vi "DAC Save Results.vi"(8 "error in":errorcluster, 9 "Log Details?":bool, 10 "tdms file":refnum<k34>, 11 "DAC Traverse in":refnum<class "DAC Traverse.lvclass">) -> (0 "error out":errorcluster)   [LabVIEW 2019, in "DAC.lvlib" / "DAC Traverse.lvclass"]
uses:
  DAC Traverse.lvclass
  DAC.lvclass
  C:/Users/krio/Documents/LV_Projects/test-stand/App/DAC/DAC.lvclass
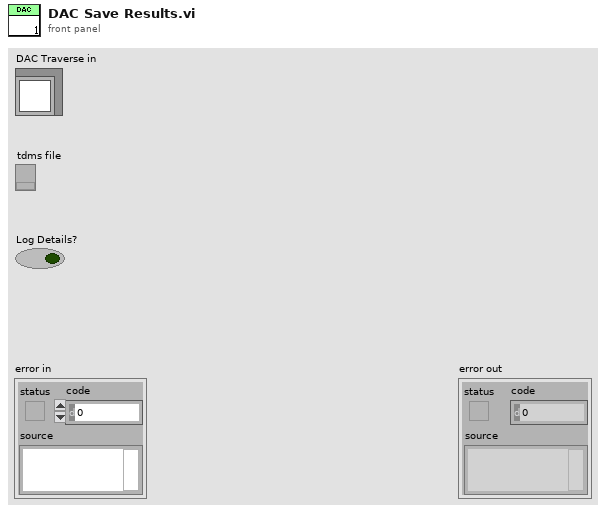
[diagram p1: front panel]
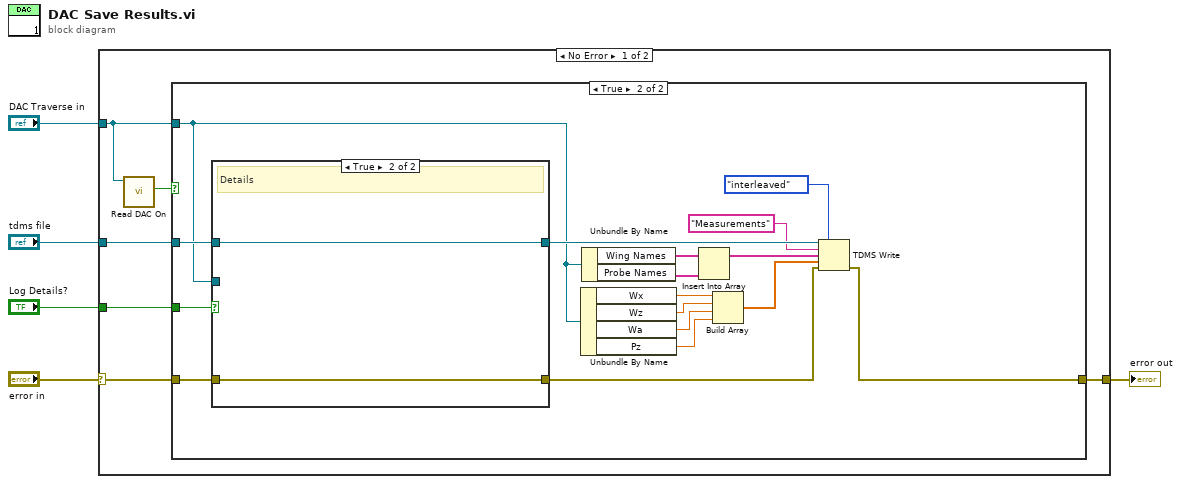
[diagram p0: block diagram]
diagram:
  n1 = case shown="No Error" "error in" {
    selector: "error in" -> [w6 w34]
    tunnel: "DAC Traverse in" -> [w11 _]
    tunnel: "tdms file" -> [w9 _]
    tunnel: [w8 w34] -> w2
    tunnel: "Log Details?" -> [w7 _]
    frame No Error {
      n2 = call "Read DAC On.vi"("DAC in"=w11) -> ("DAC On"=w10:bool)  [unwired: 8 in, 2 out]
      n3 = case shown="True" w10 {
        tunnel: w11 -> [_ w13]
        tunnel: w9 -> [_ w27]
        tunnel: [w12 w29] -> w8
        tunnel: w7 -> [_ w28]
        tunnel: w6 -> [w12 w24]
        frame False {
        }
        frame True {
          n4 = case shown="True" w28 {
            tunnel: w27 -> [w31 w33]
            tunnel: [w31 w33] -> w26
            tunnel: w13 -> [_ _]
            tunnel: w24 -> [w30 w32]
            tunnel: [w30 w32] -> w23
            frame False {
            }
            frame True {
              # "Details"
            }
          }
          n5 = Unbundle By Name(w13) -> ("Wx"=w21:dbl, "Wz"=w17:dbl, "Wa"=w16:dbl, "Pz"=w15:dbl)
          n6 = Unbundle By Name(w13) -> ("Wing Names"=w20:string[], "Probe Names"=w19:string[])
          n7 = Insert Into Array(array=w20, new element=w19) -> (w18:string[])  [unwired: 1 in]
          n8 = Build Array(w21, w17, w16, w15) -> (w14:dbl[])
          n9 = TDMS Write(0:w26, 1:enum16{"decimated", "interleaved"}."interleaved" ("data layout (0:decimated)"), 5:"Measurements" ("group name in (Untitled)"), 7:w18, 9:w14, 11:w23) -> (15:w29:errorcluster)  [unwired: 3 out]
        }
      }
    }
    frame Error {
    }
  }
  "error out" <- w2
